vi "GPS_Driver_Global.vi"() -> ()   [LabVIEW 2015]
panel:
  in  "Previous Close":dbl
  in  "Previous open":dbl
  in  "Shutter Open":dbl=2.0
  out "RODone":bool
  in  "ExpTime":dbl
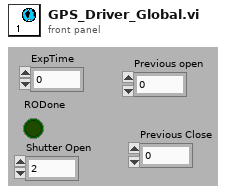
[diagram p1: front panel]
diagram:
